vi "1_5.vi"() -> ()   [LabVIEW 2020]
panel:
  out "U32":u32
  out "U8 result":u8
  out "U8 result":u8
  in  "I8":i8
  in  "U32":u32
  in  "I32":i32
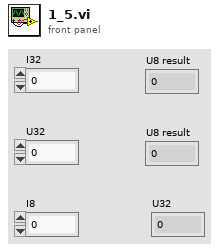
[diagram p1: front panel]
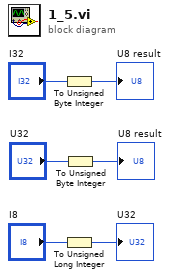
[diagram p0: block diagram]
diagram:
  n1 = To Unsigned Byte Integer(number="I32") -> (unsigned 8bit integer=→"U8 result":u8)
  n2 = To Unsigned Long Integer(number="I8") -> (unsigned 32bit integer=→"U32":u32)
  n3 = To Unsigned Byte Integer(number="U32") -> (unsigned 8bit integer=→"U8 result":u8)
